vi "PortsAnalog.vi"() -> (0 "Analog Ports":tag[](array[tag]))   [LabVIEW 2022 SP3]
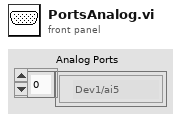
[diagram p1: front panel]
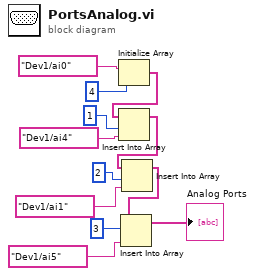
[diagram p0: block diagram]
diagram:
  n1 = Initialize Array(tag "Dev1/ai0" ("physical channels"), 4) -> (w9:tag[])
  n2 = Insert Into Array(array=w9, index=1, new element=tag "Dev1/ai4" ("physical channels")) -> (w7:tag[])
  n3 = Insert Into Array(array=w7, index=2, new element=tag "Dev1/ai1" ("physical channels")) -> (w3:tag[])
  n4 = Insert Into Array(array=w3, index=3, new element=tag "Dev1/ai5" ("physical channels")) -> (→"Analog Ports":tag[])
